vi "3HD_1BS_FPGA_v00.vi"() -> ()   [LabVIEW 2013]
doc: "Controls 6 phase locks based on the interference of two beams at a beam-splitter."
uses:
  Strict Type Defs/1BS3HD Error Signals.ctl
  Strict Type Defs/1BS3HD Lock Point.ctl
  Strict Type Defs/1BS3HD Output.ctl
  Strict Type Defs/1BS3HD Control Input.ctl
  Strict Type Defs/PII individual.ctl
  Strict Type Defs/1BS3HD Error Scale.ctl
  Strict Type Defs/1BS3HD Lock Thresh.ctl
  Strict Type Defs/1BS3HD Theta.ctl
  Strict Type Defs/Safety First.ctl
  Strict Type Defs/Scope.ctl
  Strict Type Defs/1BS3HD Max.ctl
  Strict Type Defs/1BS3HD Min.ctl
  Strict Type Defs/1BS3HD State.ctl
  <vilib>/rvi/Emulation/niFpgaSctlEmulationGetInTimedLoop.vi
  <vilib>/rvi/Emulation/niFpgaEmulationReportErrorSimple.vi
  <vilib>/rvi/Emulation/niFpgaGetClockAttributes.vi
  <vilib>/rvi/interface/RandomDataEmulation/nirviRandomDataFPGAFIFO.vi
  <vilib>/rvi/interface/RandomDataEmulation/niFpgaRandomDataHandleErrors.vi
  <vilib>/rvi/Emulation/niFpgaCriticalErrorInLSC.vi
  <vilib>/rvi/DataTransferAndStorage/Container/XNode/niFpgaContainer.xnode
  <vilib>/rvi/interface/RandomDataEmulation/nirviRandomDataFpgaReadWriteTemplate.vi
panel:
  out "State":T1
  out "Min":T2
  out "Max":T3
  in  "Graph Delay(uSec)":u32 caption="Count(uSec)"
  out "HD Errors xp":T4
  in  "Scope":T5={"Trigger Direction"=enum."plus-minus", "Delay"=0, "Aquisition Rate (Ticks)"=40, "Offset"=0, "Channel"=0, "Channel Selector"={"Channel 1"=0, "Channel 2"=4, "Channel 3"=8, "Channel 4"=8}} {"Channel Selector"."Channel 4" items=["Error Signal 1", "Error Signal 2", "Scan Trigger 1", "Scan Trigger 2", "DC Signal 1", "DC Signal 2", "PI Out 1", "PI Out 2"]; "Channel Selector"."Channel 3" items=["Error Signal 1", "Error Signal 2", "Scan Trigger 1", "Scan Trigger 2", "DC Signal 1", "DC Signal 2", "PI Out 1", "PI Out 2"]; "Channel Selector"."Channel 2" items=["Error Signal 1", "Error Signal 2", "Scan Trigger 1", "Scan Trigger 2", "DC Signal 1", "DC Signal 2", "PI Out 1", "PI Out 2"]; "Channel Selector"."Channel 1" items=["Error Signal 1", "Error Signal 2", "Scan Trigger 1", "Scan Trigger 2", "DC Signal 1", "DC Signal 2", "PI Out 1", "PI Out 2"]}
  in  "quit Control Loop":bool
  in  "Control":T6={"PII In 1"={"Lock"=FALSE, "Hold"=FALSE, "P Gain"=0, "P BS"=-5, "I Gain"=0, "I BS"=-10, "I2 G"=0, "I2 BS"=-26, "Scan Amp"=0, "Scan Off"=0, "Scan FS"=0, "SFS BS"=0, "I Max value"=10000, "I2 Max value"=10000, "Scope.Offset"=0, "Trigger Direction"=enum."either", "Scan-PII thresh"=0}, "PII In 2"={"Lock"=FALSE, "Hold"=FALSE, "P Gain"=0, "P BS"=-10, "I Gain"=0, "I BS"=-10, "I2 G"=0, "I2 BS"=-26, "Scan Amp"=0, "Scan Off"=0, "Scan FS"=0, "SFS BS"=0, "I Max value"=10000, "I2 Max value"=10000, "Scope.Offset"=0, "Trigger Direction"=enum."either", "Scan-PII thresh"=0}, "PII In 3"={"Lock"=FALSE, "Hold"=FALSE, "P Gain"=0, "P BS"=-10, "I Gain"=0, "I BS"=-10, "I2 G"=0, "I2 BS"=-26, "Scan Amp"=0, "Scan Off"=0, "Scan FS"=0, "SFS BS"=0, "I Max value"=10000, "I2 Max value"=10000, "Scope.Offset"=0, "Trigger Direction"=enum."either", "Scan-PII thresh"=0}, "Error scale"={"Pre-Offset"={"Pre-Offset 1"=2, "Pre-Offset 2"=0, "Pre-Offset 3"=0, "Pre-Offset 4"=0, "Pre-Offset 5"=2, "Pre-Offset 6"=0, "Pre-Offset 7"=2}, "Post-Offset "={"Offset 1"=0, "Offset 2"=300, "Offset 3"=0, "Offset 4"=0, "Offset 5"=0, "Offset 6"=0, "Offset 7"=0}, "Gains"={"Gain 1"=0, "Gain 2"=300, "Gain 3"=0, "Gain 4"=0, "Gain 5"=0, "Gain 6"=0, "Gain 7"=0}, "Bit Shifts"={"Bit Shift 1"=0, "Bit Shift 2"=300, "Bit Shift 3"=0, "Bit Shift 4"=0, "Bit Shift 5"=0, "Bit Shift 6"=0, "Bit Shift 7"=0}}, "Lock Thresh"={"EPR"=2, "HD A"=0, "HD B"=10, "HD C"=0}, "Re-Scan Thresh"={"EPR"=2, "HD A"=0, "HD B"=0, "HD C"=0}, "Theta"={"HD A Sin Theta"=0, "HD A Cos Theta"=0, "HD B Sin Theta"=0, "HD B Cos Theta"=0, "HD C Sin Theta"=0, "HD C Cos Theta"=0}, "Safety First"={"lim reset"=FALSE, "no limit"=FALSE, "pos slew rate * dt"=0, "neg slew rate * dt"=-10, "Hold All"=FALSE, "Count(Ticks)"=0}, "PII In 4"={"Lock"=FALSE, "Hold"=FALSE, "P Gain"=0, "P BS"=-10, "I Gain"=0, "I BS"=-10, "I2 G"=0, "I2 BS"=-26, "Scan Amp"=0, "Scan Off"=0, "Scan FS"=0, "SFS BS"=0, "I Max value"=10000, "I2 Max value"=10000, "Scope.Offset"=0, "Trigger Direction"=enum."either", "Scan-PII thresh"=0}}
  in  "\"Outputs\"":T12
  out "Outputs":T12={"EPR"=-270, "HD A"=-1710, "HD B"=880, "HD C"=0}
  in  "\"Trigger\"":T13
  out "Trigger":T13
  out "Cavity Errors":T14={"EPR"=0, "HD A"=1800, "HD B"=0, "HD C"=0}
  out "Control Loop count":i32=11285327
  out "Scope Full?":bool
  out "Scope loop count":i32=119818
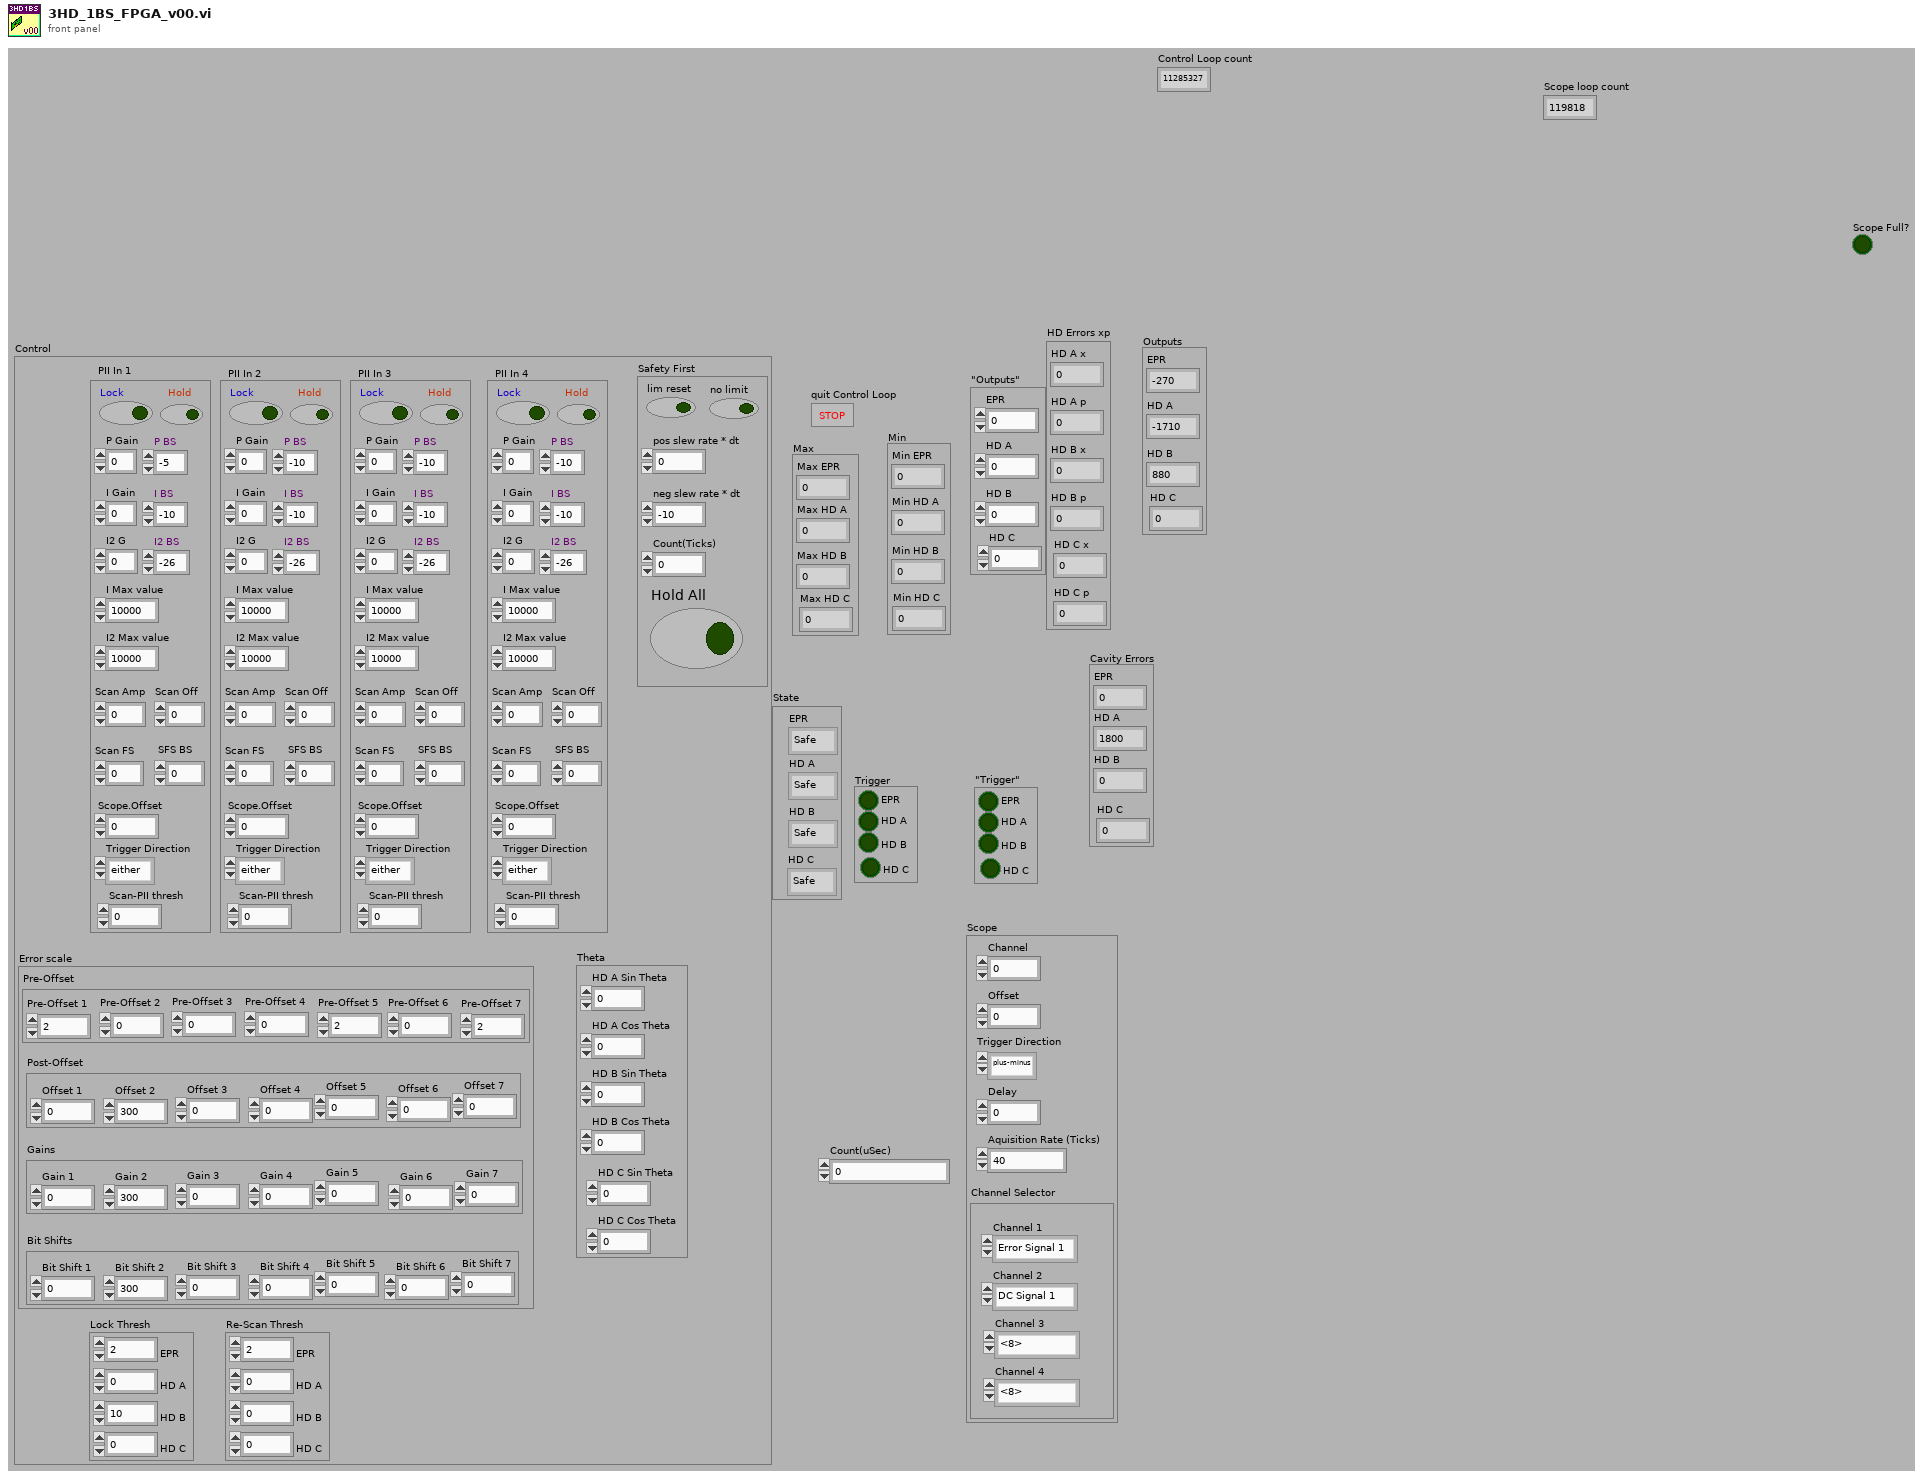
[diagram p1: front panel]
types:
  T1 = typedef "1BS3HD State.ctl" = cluster{"EPR":enum16{"Safe", "Hold", "Scan", "Lock"}, "HD A":enum16{"Safe", "Hold", "Scan", "Lock"}, "HD B":enum16{"Safe", "Hold", "Scan", "Lock"}, "HD C":enum16{"Safe", "Hold", "Scan", "Lock"}}
  T2 = typedef "1BS3HD Min.ctl" = cluster{"Min EPR":i16, "Min HD A":i16, "Min HD B":i16, "Min HD C":i16}
  T3 = typedef "1BS3HD Max.ctl" = cluster{"Max EPR":i16, "Max HD A":i16, "Max HD B":i16, "Max HD C":i16}
  T4 = cluster{"HD A x":i16, "HD A p":i16, "HD B x":i16, "HD B p":i16, "HD C p":i16, "HD C x":i16}
  T5 = typedef "Scope.ctl" = cluster{"Trigger Direction":enum8{"either", "minus-plus", "plus-minus"}, "Delay":u32, "Aquisition Rate (Ticks)":u32, "Offset":i16, "Channel":i32, "Channel Selector":cluster{"Channel 1":i32, "Channel 2":i32, "Channel 3":i32, "Channel 4":i32}}
  T6 = typedef "1BS3HD Control Input.ctl" = cluster{"PII In 1":T7, "PII In 2":T7, "PII In 3":T7, "Error scale":T8, "Lock Thresh":T9, "Re-Scan Thresh":T9, "Theta":T10, "Safety First":T11, "PII In 4":T7}
  T7 = typedef "PII individual.ctl" = cluster{"Lock":bool, "Hold":bool, "P Gain":i32, "P BS":i16, "I Gain":i32, "I BS":i16, "I2 G":i32, "I2 BS":i16, "Scan Amp":i16, "Scan Off":i16, "Scan FS":u16, "SFS BS":i16, "I Max value":i32, "I2 Max value":i32, "Scope.Offset":i16, "Trigger Direction":enum8{"either", "minus-plus", "plus-minus"}, "Scan-PII thresh":i16}
  T8 = typedef "1BS3HD Error Scale.ctl" = cluster{"Pre-Offset":cluster{"Pre-Offset 1":i16, "Pre-Offset 2":i16, "Pre-Offset 3":i16, "Pre-Offset 4":i16, "Pre-Offset 5":i16, "Pre-Offset 6":i16, "Pre-Offset 7":i16}, "Post-Offset ":cluster{"Offset 1":i16, "Offset 2":i16, "Offset 3":i16, "Offset 4":i16, "Offset 5":i16, "Offset 6":i16, "Offset 7":i16}, "Gains":cluster{"Gain 1":i16, "Gain 2":i16, "Gain 3":i16, "Gain 4":i16, "Gain 5":i16, "Gain 6":i16, "Gain 7":i16}, "Bit Shifts":cluster{"Bit Shift 1":i16, "Bit Shift 2":i16, "Bit Shift 3":i16, "Bit Shift 4":i16, "Bit Shift 5":i16, "Bit Shift 6":i16, "Bit Shift 7":i16}}
  T9 = typedef "1BS3HD Lock Thresh.ctl" = cluster{"EPR":i16, "HD A":i16, "HD B":i16, "HD C":i16}
  T10 = typedef "1BS3HD Theta.ctl" = cluster{"HD A Sin Theta":i32, "HD A Cos Theta":i32, "HD B Sin Theta":i32, "HD B Cos Theta":i32, "HD C Sin Theta":i32, "HD C Cos Theta":i32}
  T11 = typedef "Safety First.ctl" = cluster{"lim reset":bool, "no limit":bool, "pos slew rate * dt":i16, "neg slew rate * dt":i16, "Hold All":bool, "Count(Ticks)":u32}
  T12 = typedef "1BS3HD Output.ctl" = cluster{"EPR":i16, "HD A":i16, "HD B":i16, "HD C":i16}
  T13 = typedef "1BS3HD Lock Point.ctl" = cluster{"EPR":bool, "HD A":bool, "HD B":bool, "HD C":bool}
  T14 = typedef "1BS3HD Error Signals.ctl" = cluster{"EPR":i16, "HD A":i16, "HD B":i16, "HD C":i16}
  T15 = typedef "1BS3HD Signals.ctl" = cluster{"PII In 1":T7, "PII In 2":T7, "PII In 3":T7, "Lock Thresh":T9, "Re-Scan Thresh":T9, "Safety First":T11, "Graph Errors":T14, "PII In 4":T7}
  T16 = typedef "1BS3HD Control Cluster.ctl" = cluster{"Control EPR":T7, "Control HD A":T7, "Control HD B":T7, "Max":T3, "Min":T2, "Lock Threshold":T9, "Re-Scan Threshold":T9, "Lock Point?":T13, "Re-scan?":T13, "Lock pressed? (-1)":T13, "Cavity Errors":T14, "State (-1)":T1, "Safety First":T11, "Control HD C":T7}
  T17 = typedef "1BS3HD PII Scan State.ctl" = cluster{"Control EPR":T7, "Control HD A":T7, "Control HD B":T7, "Error Signals":T14, "State":T1, "Control HD C":T7}
  T18 = typedef "1BS3HD MaxMin.ctl" = cluster{"State":T1, "Reset MaxMin?":T19, "Max":T3, "Min":T2, "Lock pressed?":T13, "Safety First":T11}
  T19 = typedef "1BS3HD Reset MaxMin.ctl" = cluster{"EPR":bool, "HD A":bool, "HD B":bool, "HD C":bool}
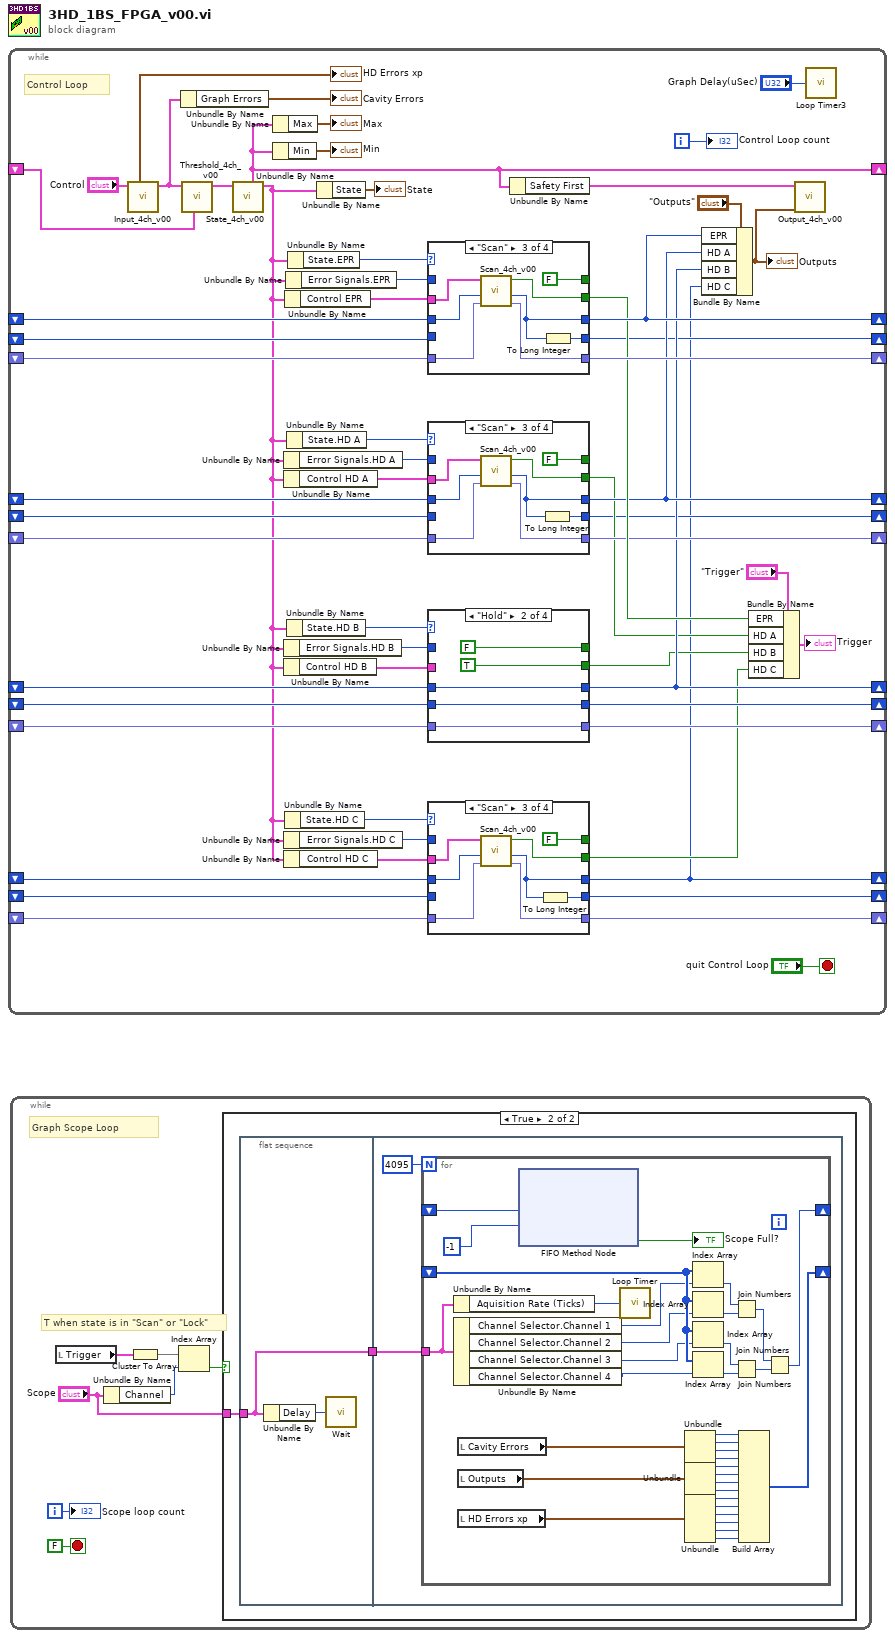
[diagram p0: block diagram]
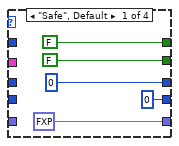
[diagram p3: hidden frame]
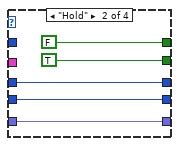
[diagram p4: hidden frame]
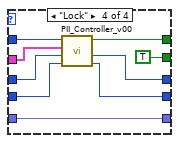
[diagram p5: hidden frame]
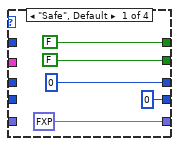
[diagram p6: hidden frame]
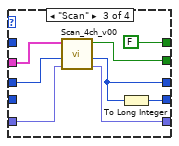
[diagram p7: hidden frame]
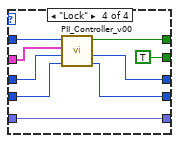
[diagram p8: hidden frame]
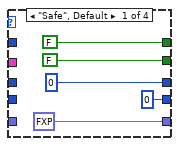
[diagram p9: hidden frame]
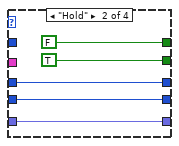
[diagram p10: hidden frame]
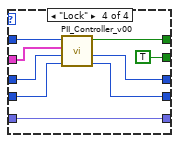
[diagram p11: hidden frame]
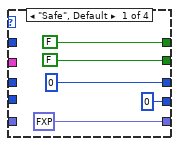
[diagram p12: hidden frame]
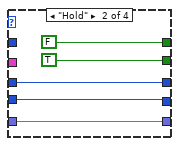
[diagram p13: hidden frame]
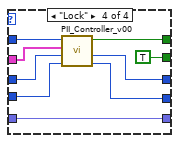
[diagram p14: hidden frame]
diagram:
  n1 = while {
    shift-right: [w29] -> _
    shift-left: _ -> [w54]
    shift-right: [w48] -> _
    shift-left: _ -> [w53]
    shift-right: [w52] -> _
    shift-left: _ -> [w51]
    shift-right: [w38] -> _
    shift-left: _ -> [w44]
    shift-right: [w43] -> _
    shift-left: _ -> [w42]
    shift-right: [w14] -> _
    shift-left: _ -> [w13]
    shift-right: [w37] -> _
    shift-left: _ -> [w39]
    shift-right: [w40] -> _
    shift-left: _ -> [w41]
    shift-right: [w18] -> _
    shift-left: _ -> [w17]
    shift-right: [w16] -> _
    shift-left: _ -> [w15]
    shift-right: [w3] -> _
    shift-left: _ -> [w9]
    shift-right: [w8] -> _
    shift-left: _ -> [w7]
    shift-right: [w6] -> _
    shift-left: _ -> [w5]
    i -> [w55]
    stop <- "quit Control Loop" stop-if-true
    # "Control Loop"
    n2 = call "Input_4ch_v00.vi"("Control"="Control") -> ("Signals"=w34:T15, "HD Errors xp"=→"HD Errors xp":T4)  [unwired: 9 in]
    n3 = Unbundle By Name(w34) -> ("Graph Errors"=→"Cavity Errors":T14)
    n4 = call "Threshold_4ch_v00.vi"("MaxMin"=w54, "Signals"=w34) -> ("Control Graph Cluster"=w31:T16)  [unwired: 9 in]
    n5 = call "State_4ch_v00.vi"("Control Cavity Cluster"=w31) -> ("PII Scan State Errors"=w2:T17, "MaxMin"=w29:T18)  [unwired: 9 in]
    n6 = Unbundle By Name(w29) -> ("Max"=→"Max":T3)
    n7 = Unbundle By Name(w29) -> ("Min"=→"Min":T2)
    n8 = Unbundle By Name(w2) -> ("Error Signals.HD A"=w23:i16)
    n9 = Unbundle By Name(w2) -> ("Control HD A"=w22:T7)
    n10 = Unbundle By Name(w2) -> ("Error Signals.HD B"=w21:i16)
    n11 = Unbundle By Name(w2) -> ("Control HD B"=w20:T7)
    n12 = Unbundle By Name(w2) -> ("Error Signals.HD C"=w12:i16)
    n13 = Unbundle By Name(w2) -> ("Control HD C"=w11:T7)
    n14 = Unbundle By Name(w2) -> ("Control EPR"=w27:T7)
    n15 = Unbundle By Name(w2) -> ("State.HD C"=w10:enum16{"Safe", "Hold", "Scan", "Lock"})
    n16 = Unbundle By Name(w2) -> ("Error Signals.EPR"=w26:i16)
    n17 = Unbundle By Name(w2) -> ("State.HD A"=w24:enum16{"Safe", "Hold", "Scan", "Lock"})
    n18 = Unbundle By Name(w2) -> ("State.HD B"=w19:enum16{"Safe", "Hold", "Scan", "Lock"})
    n19 = Unbundle By Name(w2) -> ("State.EPR"=w25:enum16{"Safe", "Hold", "Scan", "Lock"})
    n20 = Unbundle By Name(w2) -> ("State"=→"State":T1)
    n21 = case shown="\"Scan\"" w25 {
      tunnel: w26 -> [_ _ _ w167]
      tunnel: [FALSE ("I too high? (F=No)") FALSE ("I too high? (F=No)") FALSE ("I too high? (F=No)") w166] -> _
      tunnel: w27 -> [_ _ w157 w165]
      tunnel: [i16 0 ("PII out") w149 w151 w162] -> w48
      tunnel: w53 -> [_ w149 w154 w163]
      tunnel: w15 -> [_ w146 _ w159]
      tunnel: [fxp<+,33,17> 0.0 ("Scan") w148 w156 w161] -> w52
      tunnel: w51 -> [_ w148 w155 w161]
      tunnel: [FALSE ("Zero Crossing") TRUE ("Zero Crossing") w153 TRUE ("Zero Crossing")] -> w47
      tunnel: [0 ("I Cavity") w146 w152 w160] -> w16
      frame "Safe", Default {
      }
      frame "Hold" {
      }
      frame "Scan" {
        n22 = call "Scan_4ch_v00.vi"("Scan (-1)"=w155, "Scan out (-1)"=w154, "Control Cavity"=w157) -> ("Scan"=w156:fxp<+,33,17>, "Scan out"=w151:i16, "Zero Crossing"=w153:bool)  [unwired: 6 in]
        n23 = To Long Integer(number=w151) -> (32bit integer=w152:i32)
      }
      frame "Lock" {
        n24 = call "PII_Controller_v00.vi"("Integrator (-1)"=w159, "PII out (-1)"=w163, "Control Cavity"=w165, "OPO A Error"=w167) -> ("I Cavity"=w160:i32, "PII out"=w162:i16, "I too high?"=w166:bool)  [unwired: 5 in]
      }
    }
    n25 = case shown="\"Scan\"" w24 {
      tunnel: w23 -> [_ _ _ w140]
      tunnel: [FALSE ("I too high? (F=No)") FALSE ("I too high? (F=No)") FALSE ("I too high? (F=No)") w139] -> _
      tunnel: w22 -> [_ _ w130 w137]
      tunnel: [i16 0 ("PII out") w122 w124 w134] -> w38
      tunnel: w44 -> [_ w122 w127 w135]
      tunnel: w17 -> [_ w119 _ w138]
      tunnel: [fxp<+,33,17> 0.0 ("Scan") w121 w129 w133] -> w43
      tunnel: w42 -> [_ w121 w128 w133]
      tunnel: [FALSE ("Zero Crossing") TRUE ("Zero Crossing") w126 TRUE ("Zero Crossing")] -> w36
      tunnel: [0 ("I Cavity") w119 w125 w132] -> w18
      frame "Safe", Default {
      }
      frame "Hold" {
      }
      frame "Scan" {
        n26 = call "Scan_4ch_v00.vi"("Scan (-1)"=w128, "Scan out (-1)"=w127, "Control Cavity"=w130) -> ("Scan"=w129:fxp<+,33,17>, "Scan out"=w124:i16, "Zero Crossing"=w126:bool)  [unwired: 6 in]
        n27 = To Long Integer(number=w124) -> (32bit integer=w125:i32)
      }
      frame "Lock" {
        n28 = call "PII_Controller_v00.vi"("Integrator (-1)"=w138, "PII out (-1)"=w135, "Control Cavity"=w137, "OPO A Error"=w140) -> ("I Cavity"=w132:i32, "PII out"=w134:i16, "I too high?"=w139:bool)  [unwired: 5 in]
      }
    }
    n29 = case shown="\"Hold\"" w19 {
      tunnel: w21 -> [_ _ _ w113]
      tunnel: [FALSE ("I too high? (F=No)") FALSE ("I too high? (F=No)") FALSE ("I too high? (F=No)") w112] -> _
      tunnel: w20 -> [_ _ w103 w111]
      tunnel: [i16 0 ("PII out") w95 w98 w108] -> w37
      tunnel: w39 -> [_ w95 w100 w109]
      tunnel: [fxp<+,33,17> 0.0 ("Scan") w94 w102 w107] -> w40
      tunnel: w41 -> [_ w94 w101 w107]
      tunnel: [FALSE ("Zero Crossing") TRUE ("Zero Crossing") w99 TRUE ("Zero Crossing")] -> w35
      tunnel: [0 ("I Cavity") w92 w97 w106] -> w14
      tunnel: w13 -> [_ w92 _ w105]
      frame "Safe", Default {
      }
      frame "Hold" {
      }
      frame "Scan" {
        n30 = call "Scan_4ch_v00.vi"("Scan (-1)"=w101, "Scan out (-1)"=w100, "Control Cavity"=w103) -> ("Scan"=w102:fxp<+,33,17>, "Scan out"=w98:i16, "Zero Crossing"=w99:bool)  [unwired: 6 in]
        n31 = To Long Integer(number=w98) -> (32bit integer=w97:i32)
      }
      frame "Lock" {
        n32 = call "PII_Controller_v00.vi"("Integrator (-1)"=w105, "PII out (-1)"=w109, "Control Cavity"=w111, "OPO A Error"=w113) -> ("I Cavity"=w106:i32, "PII out"=w108:i16, "I too high?"=w112:bool)  [unwired: 5 in]
      }
    }
    n33 = case shown="\"Scan\"" w10 {
      tunnel: w12 -> [_ _ _ w86]
      tunnel: [FALSE ("I too high? (F=No)") FALSE ("I too high? (F=No)") FALSE ("I too high? (F=No)") w85] -> _
      tunnel: w11 -> [_ _ w76 w84]
      tunnel: [i16 0 ("PII out") w68 w71 w81] -> w3
      tunnel: w9 -> [_ w68 w73 w82]
      tunnel: [fxp<+,33,17> 0.0 ("Scan") w67 w75 w80] -> w6
      tunnel: w5 -> [_ w67 w74 w80]
      tunnel: [FALSE ("Zero Crossing") TRUE ("Zero Crossing") w72 TRUE ("Zero Crossing")] -> w4
      tunnel: [0 ("I Cavity") w65 w70 w79] -> w8
      tunnel: w7 -> [_ w65 _ w78]
      frame "Safe", Default {
      }
      frame "Hold" {
      }
      frame "Scan" {
        n34 = call "Scan_4ch_v00.vi"("Scan (-1)"=w74, "Scan out (-1)"=w73, "Control Cavity"=w76) -> ("Scan"=w75:fxp<+,33,17>, "Scan out"=w71:i16, "Zero Crossing"=w72:bool)  [unwired: 6 in]
        n35 = To Long Integer(number=w71) -> (32bit integer=w70:i32)
      }
      frame "Lock" {
        n36 = call "PII_Controller_v00.vi"("Integrator (-1)"=w78, "PII out (-1)"=w82, "Control Cavity"=w84, "OPO A Error"=w86) -> ("I Cavity"=w79:i32, "PII out"=w81:i16, "I too high?"=w85:bool)  [unwired: 5 in]
      }
    }
    n37 = Unbundle By Name(w29) -> ("Safety First"=w50:T11)
    n38 = Bundle By Name(cluster="\"Outputs\"", "EPR"=w48, "HD A"=w38, "HD B"=w37, "HD C"=w3) -> (w49:T12)
    "Outputs" <- w49
    n39 = Bundle By Name(cluster="\"Trigger\"", "EPR"=w47, "HD A"=w36, "HD B"=w35, "HD C"=w4) -> (→"Trigger":T13)
    n40 = call "Output_4ch_v00.vi"("Outputs"=w49, "Safety First"=w50) -> ()  [unwired: 10 in]
    n41 = call "Loop Timer3"("Count(uSec)"="Graph Delay(uSec)") -> ()  [unwired: 1 out]
    "Control Loop count" <- w55
  }
  n42 = while {
    i -> [w171]
    stop <- FALSE ("stop") stop-if-true
    # "Graph Scope Loop"
    # "T when state is in \"Scan\" or \"Lock\""
    n43 = local read "Trigger"() -> (w169:T13)
    n44 = Unbundle By Name("Scope") -> ("Channel"=w172:i32)
    n45 = Cluster To Array(cluster=w169) -> (array=w173:bool[])
    n46 = Index Array(array=w173, index=w172) -> (element=w170:bool)
    n47 = case shown="True" w170 {
      tunnel: "Scope" -> [_ w176]
      frame False {
      }
      frame True {
        n48 = flat-sequence {
          tunnel: w176 -> [w177]
          tunnel: [w177] -> w175
          tunnel: w175 -> [w179]
          frame #0 {
            n49 = Unbundle By Name(w177) -> ("Delay"=w178:u32)
            n50 = call "Wait"("Count(Ticks)"=w178) -> ()  [unwired: 1 out]
          }
          frame #1 {
            n51 = for {
              N: 4095 -> [_]
              tunnel: w179 -> [w214]
              shift-right: [w206] -> _
              shift-left: _ -> [w205]
              shift-right: [w201] -> _
              shift-left: _ -> [w200]
              n52 = Unbundle By Name(w214) -> ("Aquisition Rate (Ticks)"=w215:u32)
              n53 = Unbundle By Name(w214) -> ("Channel Selector.Channel 1"=w202:i32, "Channel Selector.Channel 2"=w203:i32, "Channel Selector.Channel 3"=w197:i32, "Channel Selector.Channel 4"=w204:i32)
              n54 = local read "Cavity Errors"() -> (w213:T14)
              n55 = local read "Outputs"() -> (w212:T12)
              n56 = local read "HD Errors xp"() -> (w195:T4)
              n57 = xnode ("FIFO Method Node")("Element"=w200, "Timeout"=-1) -> ("Timed Out?"=→"Scope Full?":bool)  [unwired: 1 in, 1 out]
              n58 = call "Loop Timer"("Count(uSec)"=w215) -> ()  [unwired: 1 out]
              n59 = Unbundle(w213) -> ("EPR"=w192:i16, "HD A"=w193:i16, "HD B"=w194:i16, "HD C"=w191:i16)
              n60 = Unbundle(w212) -> ("EPR"=w190:i16, "HD A"=w189:i16, "HD B"=w188:i16, "HD C"=w187:i16)
              n61 = Unbundle(w195) -> ("HD A x"=w186:i16, "HD A p"=w185:i16, "HD B x"=w184:i16, "HD B p"=w183:i16, "HD C p"=w182:i16, "HD C x"=w181:i16)
              n62 = Index Array(array=w205, index=w202) -> (element=w208:i16)
              n63 = Index Array(array=w205, index=w203) -> (element=w207:i16)
              n64 = Index Array(array=w205, index=w197) -> (element=w196:i16)
              n65 = Index Array(array=w205, index=w204) -> (element=w209:i16)
              n66 = Join Numbers(hi=w208, lo=w207) -> ((hi.lo)=w211:u32)
              n67 = Join Numbers(hi=w196, lo=w209) -> ((hi.lo)=w210:u32)
              n68 = Build Array(w192, w193, w194, w191, w190, w189, w188, w187, w186, w185, w184, w183, w182, w181) -> (w206:i16[])
              n69 = Join Numbers(hi=w211, lo=w210) -> ((hi.lo)=w201:u64)
            }
          }
        }
      }
    }
    "Scope loop count" <- w171
  }
